vi "Recording Path.vi"(8 "error in (no error)":errorcluster, 11 "TrialBasedExperiment in":refnum<class "TrialBasedExperiment.lvclass">) -> (0 "error out":errorcluster, 2 "FilePath":path, 3 "TrialBasedExperiment out":refnum<class "TrialBasedExperiment.lvclass">)   [LabVIEW 2012, in "AcquisitionCoreLibrary.lvlib" / "TrialBasedExperiment.lvclass"]
uses:
  TrialBasedExperiment.lvclass
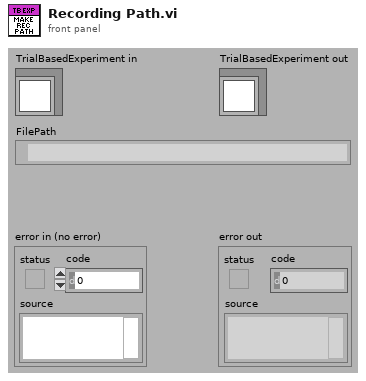
[diagram p1: front panel]
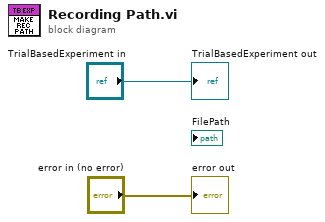
[diagram p0: block diagram]
diagram:
  "error out" <- "error in (no error)"
  "TrialBasedExperiment out" <- "TrialBasedExperiment in"
